vi "MMC_moveR.vi"(3 "Error in":errorcluster, 4 "Position Shift [counts]":i32=2000 step=1000, 5 "Axis (0..16)":i32 min=0 max=16) -> (0 "Error out":errorcluster, 2 "return":i32)   [LabVIEW 2024]
doc: "This vi moves one axis for a relative increment"
uses:
  MMC.dll
panel:
  # "MMC_moveR"
  # "Axis variable: If 0 is selected, the current active controller is used,\n if a number 1 to 16 is selected, the specified controller is activated first."
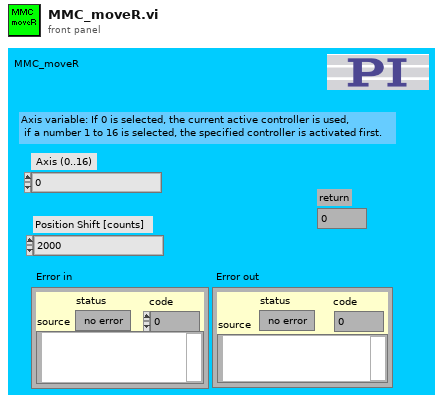
[diagram p1: front panel]
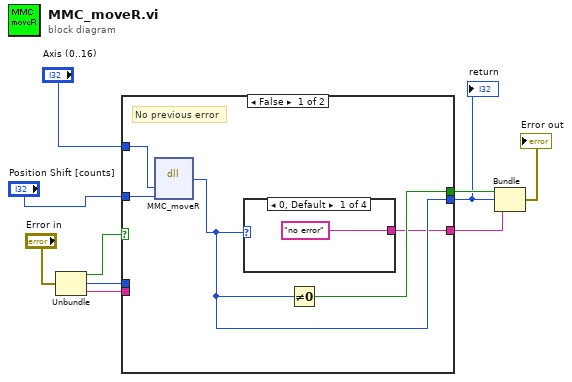
[diagram p0: block diagram]
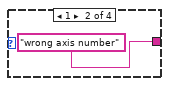
[diagram p2: hidden frame]
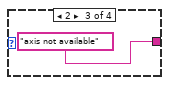
[diagram p3: hidden frame]
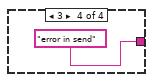
[diagram p4: hidden frame]
diagram:
  n1 = Unbundle("Error in") -> ("status"=w6:bool, "code"=w4:i32, "source"=w5:string)
  n2 = case shown="False" w6 {
    selector: w6 -> [_ w20]
    tunnel: [w15 w21] -> w1
    tunnel: [w14 w20] -> w10
    tunnel: [w13 w22] -> w8
    tunnel: w5 -> [_ w22]
    tunnel: w4 -> [_ w21]
    tunnel: "Axis (0..16)" -> [w12 _]
    tunnel: "Position Shift [counts]" -> [w11 _]
    frame False {
      # "No previous error"
      n3 = dll-call lib="E:/Wilson/HoppingSICM_TK/HoppingSICM_v1/DLLs/MMC.dll" fn="MMC_moveR"("axis"=w12, "shift"=w11) -> ("return type"=w15:i32)  [unwired: 5 in, 2 out]
      n4 = case shown="0, Default" w15 {
        tunnel: ["no error" "wrong axis number" "axis not available" "error in send"] -> w13
        frame 0, Default {
        }
        frame 1 {
        }
        frame 2 {
        }
        frame 3 {
        }
      }
      n5 = Not Equal To 0?(x=w15) -> (x != 0?=w14:bool)
    }
    frame True {
      # "error in"
    }
  }
  "return" <- w1
  n6 = Bundle(w10, "code"=w1, "source"=w8) -> (→"Error out":cluster{bool, "code":i32, "source":string})  [unwired: 1 in]
